vi "FTW-Inbox-Core-Callback.vi"(4 "Message Queue":T3 {"Routing Rules"."DropTimeout" format="%dmsec"}, 5 "Incoming Message Header":T1 {"Socket Handle" format="0x%016x"; "Header Pointer" format="0x%016x"; "Message Pointer" format="0x%016x"}, 6 "Incoming Message Event":refnum<user-event>, 7 "Common Event Data":T2) -> ()   [LabVIEW 2014]
uses:
  FTW-Inbox-Core-IncomingMessageHeader.ctl
  FTW-Inbox-Core-CallbackParameters.ctl
  json/core/FTW-JSON-Core-Structure.ctl
  FTW-Inbox-Core-RoutingRule.ctl
  json/FTW-JSON-UpdateMode.ctl
  error/FTW-ERR-ThrowGenericError.vi
  error/FTW-ERR-ThrowError.vi
  error/FTW-ERR-CallChain.vi
  string/FTW-STR-ReplaceWhitespace.vi
panel:
  out "NULL messages":i32
  out "Messages Handled":i32
  # "Inputs"
  # "Outputs"
  # "Outputs"
  # "This async callback\nhas no outputs"
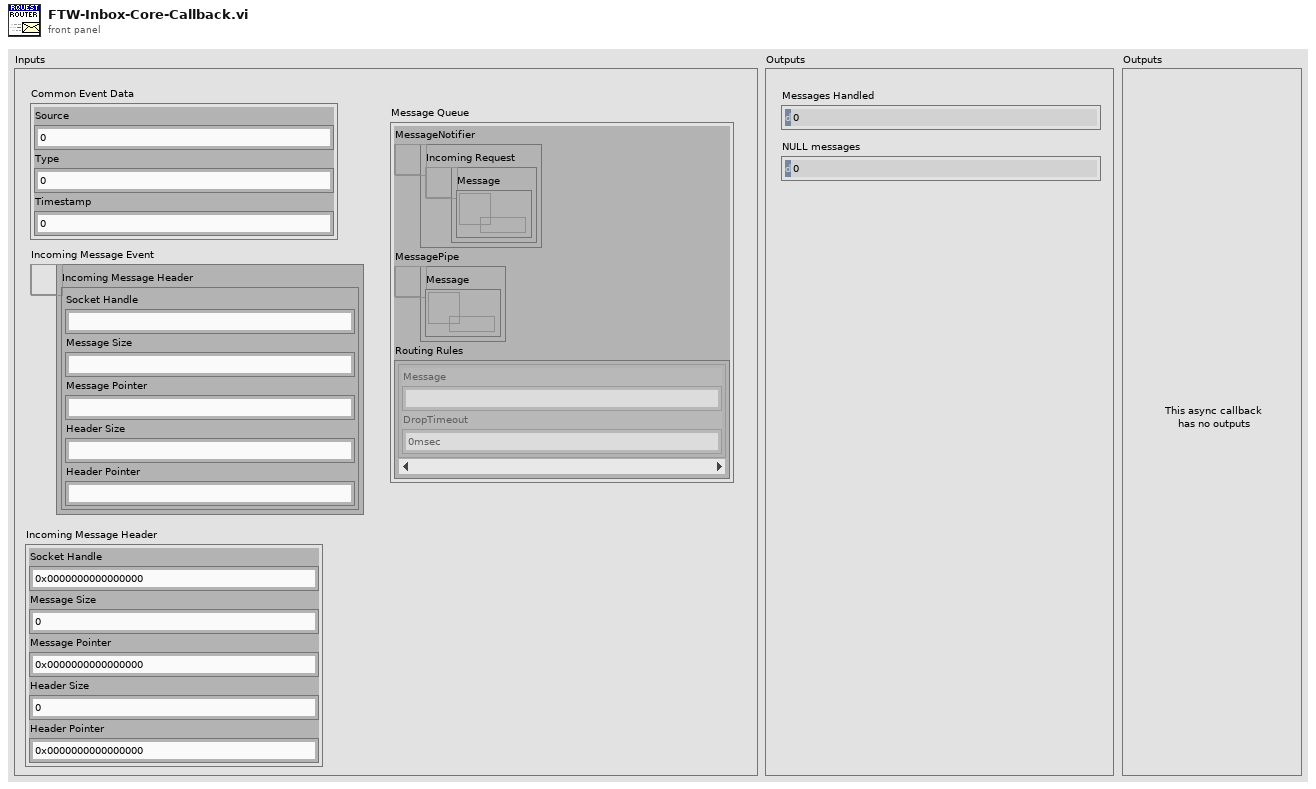
[diagram p1: front panel]
types:
  T1 = typedef "FTW-Inbox-Core-IncomingMessageHeader.ctl" = cluster{"Socket Handle":i64, "Message Size":i64, "Message Pointer":i64, "Header Size":i64, "Header Pointer":i64}
  T2 = cluster{"Source":u32, "Type":u32, "Timestamp":u32}
  T3 = typedef "FTW-Inbox-Core-CallbackParameters.ctl" = cluster{"MessageNotifier":refnum<user-event>, "MessagePipe":refnum<queue>, "Routing Rules":T4[]}
  T4 = typedef "FTW-Inbox-Core-RoutingRule.ctl" = cluster{"Message":string, "DropTimeout":i32}
  T5 = typedef "FTW-JSON-UpdateMode.ctl" = enum32{"Upsert", "Update Only", "Insert Only"}
  T6 = typedef "FTW-JSON-Core-Structure.ctl" = cluster{"JSON Object":i64, "Encoding Flags":i64, "Decoding Flags":i64}
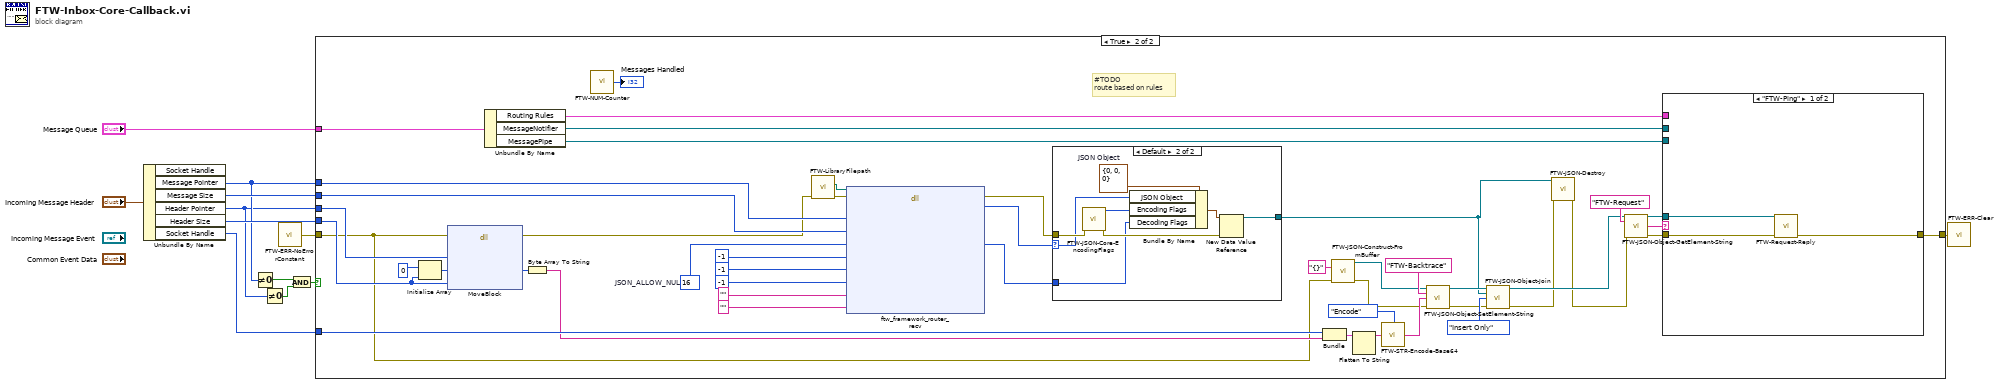
[diagram p0: block diagram]
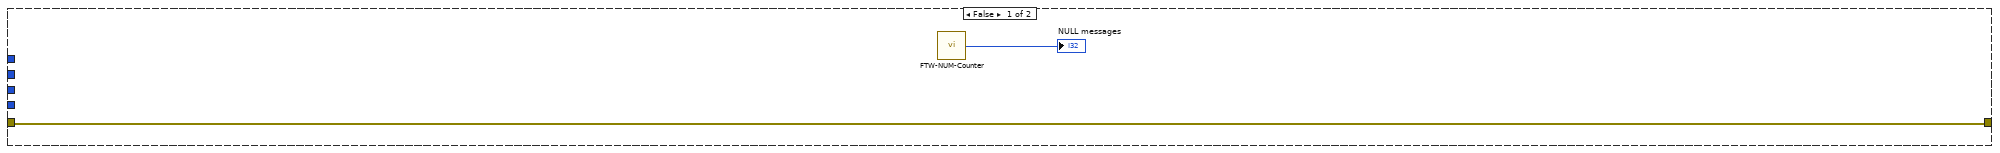
[diagram p2: hidden frame]
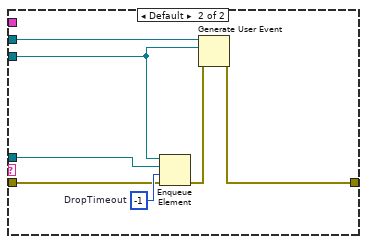
[diagram p3: hidden frame]
diagram:
  n1 = Unbundle By Name("Incoming Message Header") -> ("Message Pointer"=w7:i64, "Message Size"=w11:i64, "Header Pointer"=w6:i64, "Header Size"=w10:i64, "Socket Handle"=w1:i64)  [unwired: 1 out]
  n2 = Not Equal To 0?(x=w7) -> (x != 0?=w4:bool)
  n3 = Not Equal To 0?(x=w6) -> (x != 0?=w3:bool)
  n4 = call "FTW-ERR-NoErrorConstant.vi"() -> ("no error"=w2:errorcluster)
  n5 = And(x=w4, y=w3) -> (x .and. y?=w5:bool)
  n6 = case shown="True" w5 {
    tunnel: [w13 w61] -> w12
    tunnel: w7 -> [_ w23]
    tunnel: w11 -> [_ w22]
    tunnel: w6 -> [_ w60]
    tunnel: w10 -> [_ w51]
    tunnel: "Message Queue" -> [_ w58]
    tunnel: w1 -> [_ w44]
    tunnel: w2 -> [w13 w16]
    frame False {
      n7 = call "FTW-NUM-Counter.vi"() -> ("Counter"=→"NULL messages":i32)  [unwired: 1 in]
    }
    frame True {
      w21 = i64 16  # JSON_ALLOW_NUL
      # "#TODO\nroute based on rules"
      n8 = Initialize Array(u8 0, w51) -> (w52:u8[])
      n9 = dll-call lib="LabVIEW" fn="MoveBlock"(error in=w16, "Source Pointer"=w60, "Destination"=w52, "Length"=w51) -> (error out=w15:errorcluster, "Destination"=w59:u8[])  [unwired: 5 in, 1 out]
      n10 = Unbundle By Name(w58) -> ("Routing Rules"=w54:T4[], "MessageNotifier"=w56:refnum<user-event>, "MessagePipe"=w55:refnum<queue>)
      n11 = Byte Array To String(unsigned byte array=w59) -> (string=w43:string)
      n12 = call "FTW-NUM-Counter.vi"() -> ("Counter"=→"Messages Handled":i32)  [unwired: 1 in]
      n13 = call "FTW-LibraryFilepath.vi"("error in"=w15) -> ("error out"=w20:errorcluster, "Library Filepath"=w24:path)  [unwired: 8 in, 1 out]
      n14 = dll-call lib="?" fn="ftw_framework_router_recv"(path in=w24, error in=w20, "Message"=w23, "Message Length"=w22, "Flags"=w21, "Error Line Number"=i64 -1, "Error Column Number"=i64 -1, "Error Byte Position"=i64 -1, "Error Source"="", "Error Hint"="") -> (error out=w17:errorcluster, "JSON Object Pointer"=w19:i64, "Flags"=w18:i64)  [unwired: 8 in, 1 out]
      n15 = case shown="Default" w19 {
        selector: w19 -> [_ w72]
        tunnel: [_ w75] -> w32
        tunnel: w17 -> [_ w74]
        tunnel: w18 -> [_ w73]
        frame 0 {
        }
        frame Default {
          w76 = T6 {"JSON Object"=0, "Encoding Flags"=0, "Decoding Flags"=0}  # JSON Object
          n16 = call "FTW-JSON-Core-EncodingFlags.vi"("error in"=w74) -> ("Encoding Flags"=w78:i64, "error out"=w79:errorcluster)  [unwired: 13 in]
          n17 = Bundle By Name(cluster=w76, "JSON Object"=w72, "Encoding Flags"=w78, "Decoding Flags"=w73) -> (w77:T6)
          n18 = New Data Value Reference(data value=w77, error in=w79) -> (data value reference=w75:refnum<data-value>)  [unwired: 1 out]
        }
      }
      n19 = Bundle("Socket Handle"=w44, "string"=w43) -> (w45:cluster{"Socket Handle":i64, "string":string})  [unwired: 1 in]
      n20 = call "FTW-JSON-Construct-FromBuffer.vi"("JSON String (UTF-8)"="{}", "error in"=w16) -> ("JSON Object"=w40:refnum<data-value>, "error out"=w39:errorcluster)  [unwired: 12 in]
      n21 = Flatten To String(anything=w45) -> (data string=w46:string)  [unwired: 3 in, 2 out]
      n22 = call "FTW-STR-Encode-Base64.vi"("Input"=w46, "Direction"=enum16{"Encode", "Decode"}."Encode") -> ("Output"=w41:string)
      n23 = call "FTW-JSON-Object-SetElement-String.vi"("JSON Object"=w40, "Key"="FTW-Backtrace", "Value"=w41, "error in"=w39) -> ("JSON Object out"=w37:refnum<data-value>, "error out"=w35:errorcluster)  [unwired: 10 in]
      n24 = call "FTW-JSON-Object-Join.vi"("JSON Object"=w37, "JSON Object to Merge"=w32, "Join Mode"=FTW-JSON-UpdateMode."Insert Only", "error in"=w35) -> ("JSON Object out"=w33:refnum<data-value>, "error out"=w31:errorcluster)  [unwired: 10 in]
      n25 = call "FTW-JSON-Destroy.vi"("JSON Object"=w32, "error in"=w31) -> ("error out"=w30:errorcluster)  [unwired: 13 in]
      n26 = call "FTW-JSON-Object-GetElement-String.vi"("JSON Object"=w33, "Key"="FTW-Request", "error in"=w30) -> ("JSON Object out"=w34:refnum<data-value>, "Value"=w48:string, "error out"=w49:errorcluster)  [unwired: 9 in, 1 out]
      n27 = case shown="\"FTW-Ping\"" w48 {
        tunnel: [w62 w71] -> w61
        tunnel: w49 -> [w63 w65]
        tunnel: w56 -> [_ w70]
        tunnel: w55 -> [_ w67]
        tunnel: w54 -> [_ _]
        tunnel: w34 -> [w64 w66]
        frame "FTW-Ping" {
          n28 = call "FTW-Request-Reply.vi"("Request"=w64, "error in"=w63) -> ("error out"=w62:errorcluster)  [unwired: 13 in]
        }
        frame Default {
          w68 = -1  # DropTimeout
          n29 = Enqueue Element(queue=w67, element=w66, timeout in ms (-1)=w68, error in (no error)=w65) -> (error out=w69:errorcluster)  [unwired: 2 out]
          n30 = Generate User Event(user event=w70, event data cluster=w67, error in=w69) -> (error out=w71:errorcluster)  [unwired: 1 in, 1 out]
        }
      }
    }
  }
  n31 = call "FTW-ERR-Clear.vi"("error to snuff"=w12) -> ()  [unwired: 1 out]
